vi "Open-close-Gate.vi"() -> ()   [LabVIEW 2013]
panel:
  in  "StopProgram":bool
  in  "LowVacuum":dbl
  out "Fore_Samp":bool
  out "Samp_Atmos":bool
  in  "Tar. In":bool
  out "LenseHVSet":dbl
  out "PulseHVSet":dbl
  out "TarHVSet":dbl
  out "MCPHVSet":dbl
  in  "LenseHV":dbl
  in  "PulseHV":dbl
  in  "TarHV":dbl
  in  "MCPHV":dbl
  in  "ConfiguredPumpCom":refnum<visa-resource-name>
  in  "TakeMS_Run":bool
  in  "Laseron":bool
  in  "OpenCloseGate":bool
  # "FromPanel"
  # "Laser RS232"
  # "Get DI"
  # "GetAI"
  # "SetAO"
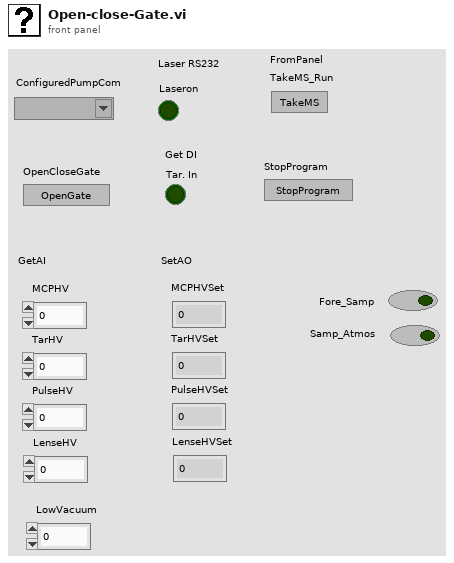
[diagram p1: front panel]
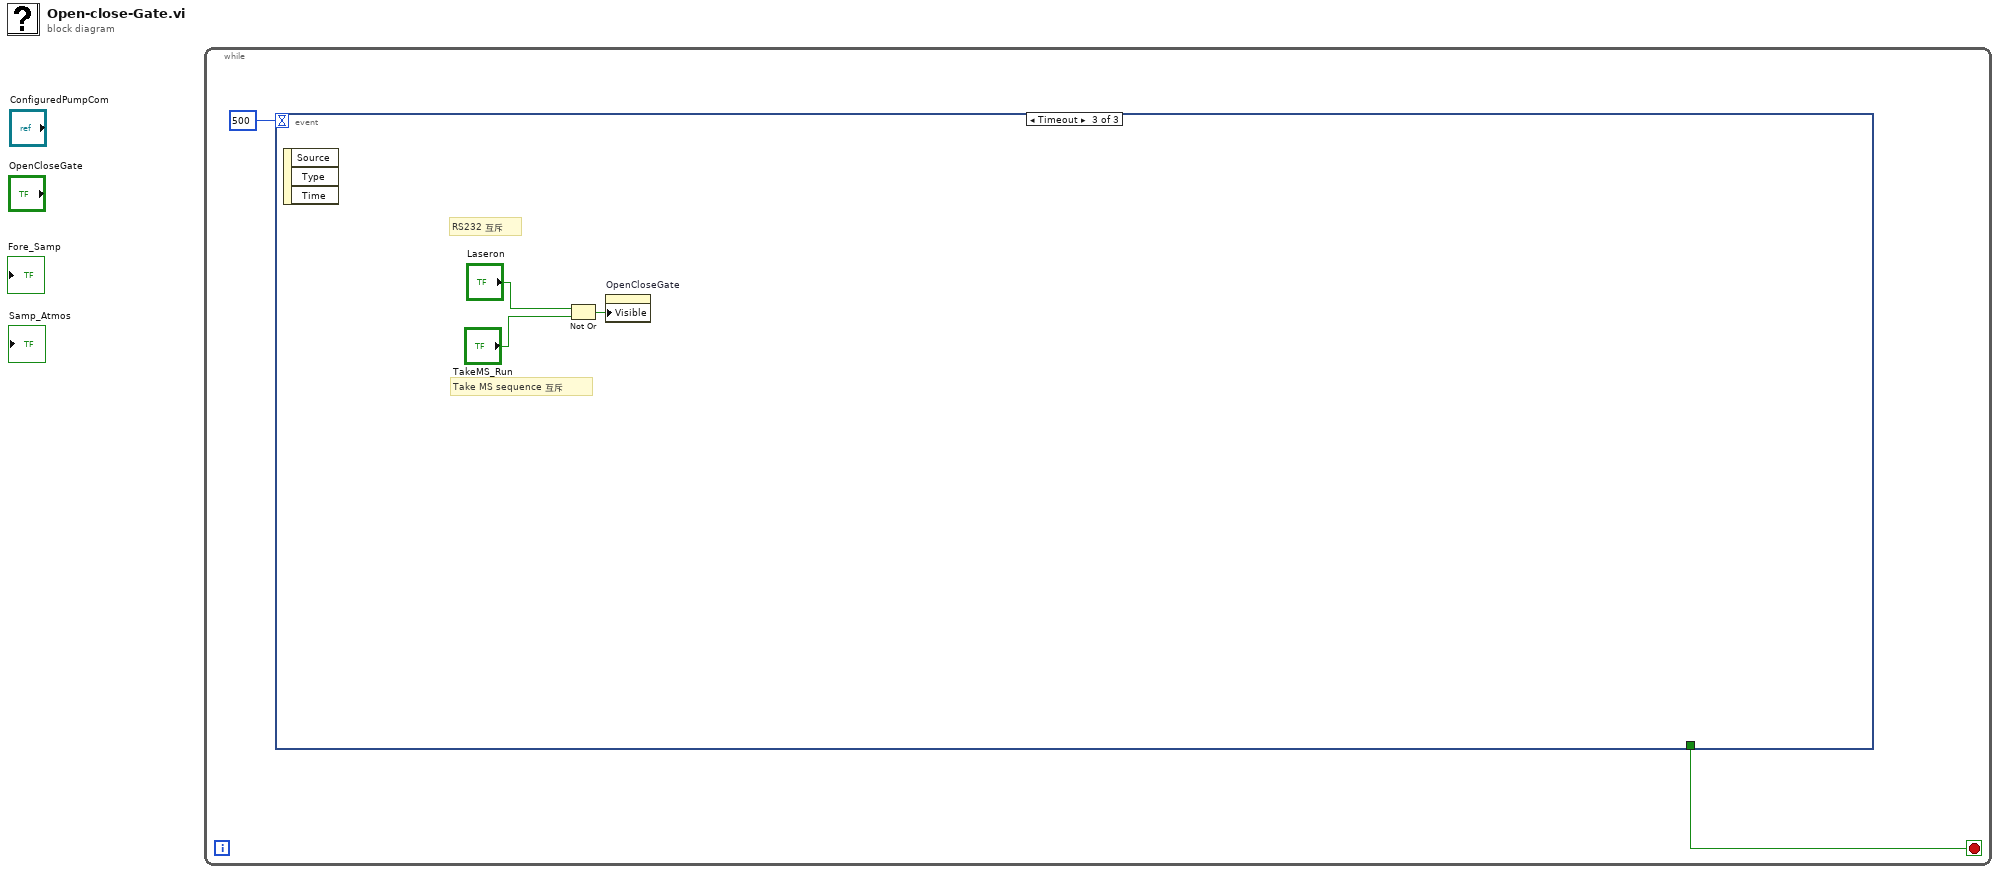
[diagram p0: block diagram]
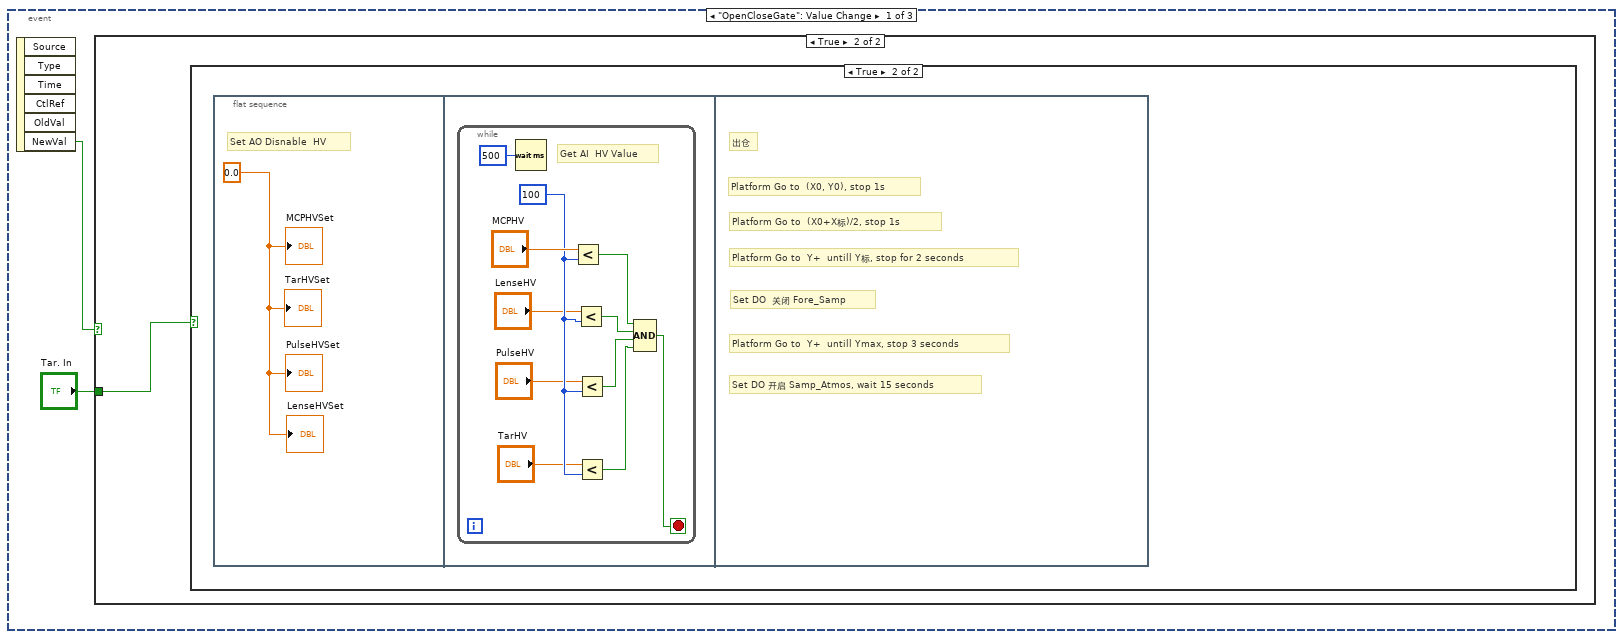
[diagram p2: hidden frame]
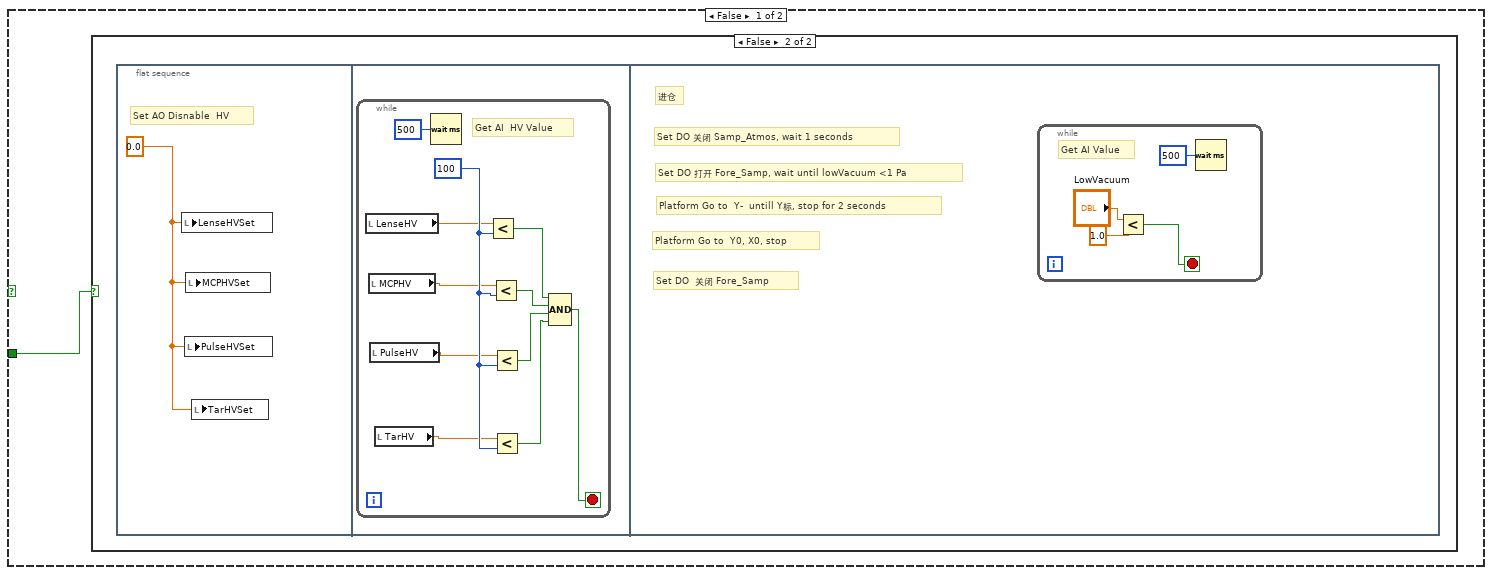
[diagram p3: hidden frame]
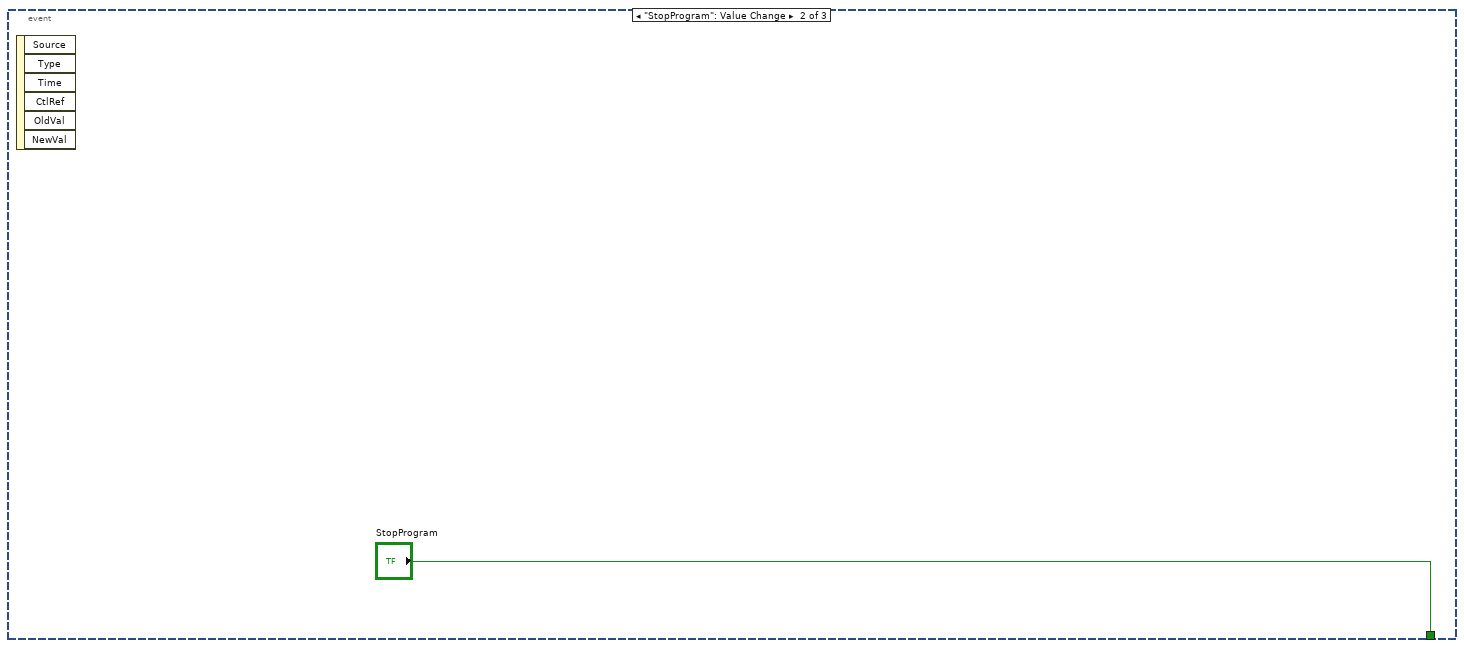
[diagram p6: hidden frame]
diagram:
  n1 = while {
    stop <- w1 stop-if-true
    n2 = event shown="[2] Timeout" {
      selector: _ -> [_ _ _]
      dyn-events: _ -> [_ _ _]
      timeout: 500 -> [_ _ _]
      tunnel: [_ "StopProgram" _] -> w1
      event "OpenCloseGate": Value Change {
        n3 = event-data() -> ("NewVal"=w4:bool)  [unwired: 1 in, 5 out]
        n4 = case shown="True" w4 {
          tunnel: "Tar. In" -> [w5 w22]
          frame False {
            n5 = case shown="False" w5 {
              frame True {
              }
              frame False {
                n6 = flat-sequence {
                  frame #0 {
                    w6 = 0.0 ("MCPHVSet")
                    # "Set AO Disnable  HV"
                    n7 = local write "LenseHVSet"(w6) -> ()
                    n8 = local write "PulseHVSet"(w6) -> ()
                    n9 = local write "MCPHVSet"(w6) -> ()
                    n10 = local write "TarHVSet"(w6) -> ()
                  }
                  frame #1 {
                    n11 = while {
                      stop <- w11 stop-if-true
                      w16 = 100
                      # "Get AI  HV Value"
                      n12 = local read "LenseHV"() -> (w10:dbl)
                      n13 = local read "MCPHV"() -> (w9:dbl)
                      n14 = local read "PulseHV"() -> (w8:dbl)
                      n15 = local read "TarHV"() -> (w7:dbl)
                      n16 = Wait (ms)(milliseconds to wait=u32 500) -> ()  [unwired: 1 out]
                      n17 = Less?(x=w10, y=w16) -> (x < y?=w15:bool)
                      n18 = Less?(x=w9, y=w16) -> (x < y?=w14:bool)
                      n19 = Less?(x=w8, y=w16) -> (x < y?=w13:bool)
                      n20 = Less?(x=w7, y=w16) -> (x < y?=w12:bool)
                      n21 = Compound Arithmetic op=AND(w15, w14, w13, w12) -> (w11:bool)
                    }
                  }
                  frame #2 {
                    # "进仓"
                    # "Set DO 打开 Fore_Samp, wait until lowVacuum <1 Pa"
                    # "Set DO 关闭 Samp_Atmos, wait 1 seconds"
                    # "Set DO  关闭 Fore_Samp"
                    # "Platform Go to  Y-  untill Y标, stop for 2 seconds"
                    # "Platform Go to  Y0, X0, stop"
                    n22 = while {
                      stop <- w19 stop-if-true
                      # "Get AI Value"
                      n23 = Less?(x="LowVacuum", y=1.0) -> (x < y?=w19:bool)
                      n24 = Wait (ms)(milliseconds to wait=u32 500) -> ()  [unwired: 1 out]
                    }
                  }
                }
              }
            }
          }
          frame True {
            n25 = case shown="True" w22 {
              frame False {
              }
              frame True {
                n26 = flat-sequence {
                  frame #0 {
                    w23 = 0.0 ("MCPHVSet")
                    # "Set AO Disnable  HV"
                    "MCPHVSet" <- w23
                    "TarHVSet" <- w23
                    "PulseHVSet" <- w23
                    "LenseHVSet" <- w23
                  }
                  frame #1 {
                    n27 = while {
                      stop <- w24 stop-if-true
                      w32 = 100
                      # "Get AI  HV Value"
                      n28 = Wait (ms)(milliseconds to wait=u32 500) -> ()  [unwired: 1 out]
                      n29 = Less?(x="MCPHV", y=w32) -> (x < y?=w28:bool)
                      n30 = Less?(x="LenseHV", y=w32) -> (x < y?=w27:bool)
                      n31 = Less?(x="PulseHV", y=w32) -> (x < y?=w26:bool)
                      n32 = Less?(x="TarHV", y=w32) -> (x < y?=w25:bool)
                      n33 = Compound Arithmetic op=AND(w28, w27, w26, w25) -> (w24:bool)
                    }
                  }
                  frame #2 {
                    # "出仓"
                    # "Platform Go to  (X0, Y0), stop 1s"
                    # "Set DO 开启 Samp_Atmos, wait 15 seconds"
                    # "Set DO  关闭 Fore_Samp"
                    # "Platform Go to  Y+  untill Ymax, stop 3 seconds"
                    # "Platform Go to  Y+  untill Y标, stop for 2 seconds"
                    # "Platform Go to  (X0+X标)/2, stop 1s"
                  }
                }
              }
            }
          }
        }
      }
      event "StopProgram": Value Change {
        n34 = event-data() -> ()  [unwired: 1 in, 6 out]
      }
      event Timeout {
        # "Take MS sequence 互斥"
        # "RS232 互斥"
        n35 = event-data() -> ()  [unwired: 1 in, 3 out]
        n36 = Not Or(1:"TakeMS_Run", 2:"Laseron") -> (0:w38:bool)
        n37 = property on="OpenCloseGate" class="Bool (strict)"("Visible"=w38) -> ()  [unwired: 2 in, 2 out]
      }
    }
  }
